vi "Initialize Custom Device.vi"(8 "error in":errorcluster, 11 "Ballard MIL-STD 1553 in":T1=18446744073709551615 format="%.0x") -> (0 "error out":errorcluster, 3 "Ballard MIL-STD 1553 out":T1 format="%.0x")   [LabVIEW 2020, in "Ballard MIL-STD-1553 Scripting.lvlib"]
uses:
  Ballard MIL-STD-1553 Scripting.lvlib
  <vilib>/NI VeriStand/Custom Device API/Custom Device Item Ref.ctl
  <vilib>/NI VeriStand/Custom Device API/Custom Device API.lvlib
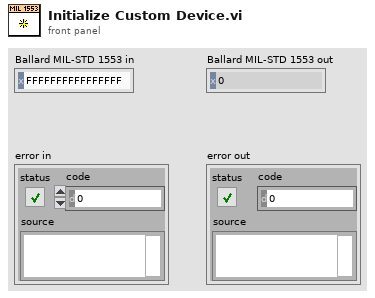
[diagram p1: front panel]
types:
  T1 = typedef "Custom Device API.lvlib/Custom Device Item Ref.ctl" = u64
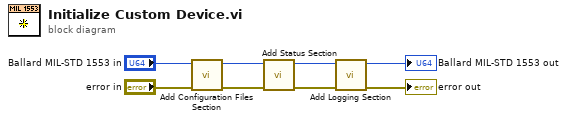
[diagram p0: block diagram]
diagram:
  n1 = call "Add Configuration Files Section.vi"("error in"="error in", "custom device in"="Ballard MIL-STD 1553 in") -> ("error out"=w5:errorcluster, "custom device out"=w6:T1)  [unwired: 7 in, 1 out]
  n2 = call "Add Status Section.vi"("error in"=w5, "custom device in"=w6) -> ("error out"=w4:errorcluster, "custom device out"=w3:T1)  [unwired: 7 in, 1 out]
  n3 = call "Add Logging Section.vi"("error in"=w4, "Ballard ARINC 429 custom device in"=w3) -> ("error out"=→"error out":errorcluster, "Ballard ARINC 429 custom device out"=→"Ballard MIL-STD 1553 out":T1)  [unwired: 7 in, 1 out]
